vi "Auto Drive.vi"(0 "Ticks(Distance)":dbl=978.0 format="%#_13g", 1 "Swerve DevRef":T2[](array[typedef])=[{"DeviceStatus"={"status"=FALSE, "code"=0, "source"=""}, "Type"=enum."CAN", "PWM"={"PWM Channel"=enum."PWM 1", "DeadBand"={"Name"="", "maxPositivePwm"=0, "minPositivePwm"=0, "centerPwm"=0, "maxNegativePwm"=0, "minNegativePwm"=0, "angularRange"=0}}, "CAN"={"Device Number"=4, "SetOutput VI Ref"=variant(refnum<vi> refnum), "GetOutput VI Ref"=variant(refnum<vi> refnum), "Enable VI Ref"=variant(refnum<vi> refnum), "Disable VI Ref"=variant(refnum<vi> refnum), "Data"=variant(cluster{"Control Mode":enum8{"Percent VBus", "Speed", "Position", "Slave", "Unchanged / Invalid", "Voltage Compensation", "Current", "Motion Profile", "Motion Magic"}, "Encoder Initial Position":dbl, "MaxVout":dbl} {"Control Mode"=enum."Position", "Encoder Initial Position"=0.0, "MaxVout"=12.0})}, "Invert"=FALSE}, {"DeviceStatus"={"status"=FALSE, "code"=0, "source"=""}, "Type"=enum."CAN", "PWM"={"PWM Channel"=enum."PWM 1", "DeadBand"={"Name"="", "maxPositivePwm"=0, "minPositivePwm"=0, "centerPwm"=0, "maxNegativePwm"=0, "minNegativePwm"=0, "angularRange"=0}}, "CAN"={"Device Number"=8, "SetOutput VI Ref"=variant(refnum<vi> refnum), "GetOutput VI Ref"=variant(refnum<vi> refnum), "Enable VI Ref"=variant(refnum<vi> refnum), "Disable VI Ref"=variant(refnum<vi> refnum), "Data"=variant(cluster{"Control Mode":enum8{"Percent VBus", "Speed", "Position", "Slave", "Unchanged / Invalid", "Voltage Compensation", "Current", "Motion Profile", "Motion Magic"}, "Encoder Initial Position":dbl, "MaxVout":dbl} {"Control Mode"=enum."Position", "Encoder Initial Position"=0.0, "MaxVout"=12.0})}, "Invert"=FALSE}, {"DeviceStatus"={"status"=FALSE, "code"=0, "source"=""}, "Type"=enum."CAN", "PWM"={"PWM Channel"=enum."PWM 1", "DeadBand"={"Name"="", "maxPositivePwm"=0, "minPositivePwm"=0, "centerPwm"=0, "maxNegativePwm"=0, "minNegativePwm"=0, "angularRange"=0}}, "CAN"={"Device Number"=6, "SetOutput VI Ref"=variant(refnum<vi> refnum), "GetOutput VI Ref"=variant(refnum<vi> refnum), "Enable VI Ref"=variant(refnum<vi> refnum), "Disable VI Ref"=variant(refnum<vi> refnum), "Data"=variant(cluster{"Control Mode":enum8{"Percent VBus", "Speed", "Position", "Slave", "Unchanged / Invalid", "Voltage Compensation", "Current", "Motion Profile", "Motion Magic"}, "Encoder Initial Position":dbl, "MaxVout":dbl} {"Control Mode"=enum."Position", "Encoder Initial Position"=0.0, "MaxVout"=12.0})}, "Invert"=FALSE}, {"DeviceStatus"={"status"=FALSE, "code"=0, "source"=""}, "Type"=enum."CAN", "PWM"={"PWM Channel"=enum."PWM 1", "DeadBand"={"Name"="", "maxPositivePwm"=0, "minPositivePwm"=0, "centerPwm"=0, "maxNegativePwm"=0, "minNegativePwm"=0, "angularRange"=0}}, "CAN"={"Device Number"=2, "SetOutput VI Ref"=variant(refnum<vi> refnum), "GetOutput VI Ref"=variant(refnum<vi> refnum), "Enable VI Ref"=variant(refnum<vi> refnum), "Disable VI Ref"=variant(refnum<vi> refnum), "Data"=variant(cluster{"Control Mode":enum8{"Percent VBus", "Speed", "Position", "Slave", "Unchanged / Invalid", "Voltage Compensation", "Current", "Motion Profile", "Motion Magic"}, "Encoder Initial Position":dbl, "MaxVout":dbl} {"Control Mode"=enum."Position", "Encoder Initial Position"=0.0, "MaxVout"=12.0})}, "Invert"=FALSE}], 5 "Drive Angle":dbl=3.141592653589793, 7 "Start Power":dbl=0.2 format="%#_13g", 9 "Time Condition":u32=15000, 11 "error in":errorcluster, 12 "Wheel DevRef":T2[](array[typedef])=[{"DeviceStatus"={"status"=FALSE, "code"=0, "source"=""}, "Type"=enum."CAN", "PWM"={"PWM Channel"=enum."PWM 1", "DeadBand"={"Name"="", "maxPositivePwm"=0, "minPositivePwm"=0, "centerPwm"=0, "maxNegativePwm"=0, "minNegativePwm"=0, "angularRange"=0}}, "CAN"={"Device Number"=3, "SetOutput VI Ref"=variant(refnum<vi> refnum), "GetOutput VI Ref"=variant(refnum<vi> refnum), "Enable VI Ref"=variant(refnum<vi> refnum), "Disable VI Ref"=variant(refnum<vi> refnum), "Data"=variant(cluster{"Control Mode":enum8{"Percent VBus", "Speed", "Position", "Slave", "Unchanged / Invalid", "Voltage Compensation", "Current", "Motion Profile", "Motion Magic"}, "Encoder Initial Position":dbl, "MaxVout":dbl} {"Control Mode"=enum."Percent VBus", "Encoder Initial Position"=0.0, "MaxVout"=12.0})}, "Invert"=TRUE}, {"DeviceStatus"={"status"=FALSE, "code"=0, "source"=""}, "Type"=enum."CAN", "PWM"={"PWM Channel"=enum."PWM 1", "DeadBand"={"Name"="", "maxPositivePwm"=0, "minPositivePwm"=0, "centerPwm"=0, "maxNegativePwm"=0, "minNegativePwm"=0, "angularRange"=0}}, "CAN"={"Device Number"=7, "SetOutput VI Ref"=variant(refnum<vi> refnum), "GetOutput VI Ref"=variant(refnum<vi> refnum), "Enable VI Ref"=variant(refnum<vi> refnum), "Disable VI Ref"=variant(refnum<vi> refnum), "Data"=variant(cluster{"Control Mode":enum8{"Percent VBus", "Speed", "Position", "Slave", "Unchanged / Invalid", "Voltage Compensation", "Current", "Motion Profile", "Motion Magic"}, "Encoder Initial Position":dbl, "MaxVout":dbl} {"Control Mode"=enum."Percent VBus", "Encoder Initial Position"=0.0, "MaxVout"=12.0})}, "Invert"=TRUE}, {"DeviceStatus"={"status"=FALSE, "code"=0, "source"=""}, "Type"=enum."CAN", "PWM"={"PWM Channel"=enum."PWM 1", "DeadBand"={"Name"="", "maxPositivePwm"=0, "minPositivePwm"=0, "centerPwm"=0, "maxNegativePwm"=0, "minNegativePwm"=0, "angularRange"=0}}, "CAN"={"Device Number"=5, "SetOutput VI Ref"=variant(refnum<vi> refnum), "GetOutput VI Ref"=variant(refnum<vi> refnum), "Enable VI Ref"=variant(refnum<vi> refnum), "Disable VI Ref"=variant(refnum<vi> refnum), "Data"=variant(cluster{"Control Mode":enum8{"Percent VBus", "Speed", "Position", "Slave", "Unchanged / Invalid", "Voltage Compensation", "Current", "Motion Profile", "Motion Magic"}, "Encoder Initial Position":dbl, "MaxVout":dbl} {"Control Mode"=enum."Percent VBus", "Encoder Initial Position"=0.0, "MaxVout"=12.0})}, "Invert"=FALSE}, {"DeviceStatus"={"status"=FALSE, "code"=0, "source"=""}, "Type"=enum."CAN", "PWM"={"PWM Channel"=enum."PWM 1", "DeadBand"={"Name"="", "maxPositivePwm"=0, "minPositivePwm"=0, "centerPwm"=0, "maxNegativePwm"=0, "minNegativePwm"=0, "angularRange"=0}}, "CAN"={"Device Number"=1, "SetOutput VI Ref"=variant(refnum<vi> refnum), "GetOutput VI Ref"=variant(refnum<vi> refnum), "Enable VI Ref"=variant(refnum<vi> refnum), "Disable VI Ref"=variant(refnum<vi> refnum), "Data"=variant(cluster{"Control Mode":enum8{"Percent VBus", "Speed", "Position", "Slave", "Unchanged / Invalid", "Voltage Compensation", "Current", "Motion Profile", "Motion Magic"}, "Encoder Initial Position":dbl, "MaxVout":dbl} {"Control Mode"=enum."Percent VBus", "Encoder Initial Position"=0.0, "MaxVout"=12.0})}, "Invert"=FALSE}]) -> (15 "error out":errorcluster)   [LabVIEW 2016]
uses:
  <vilib>/Rock Robotics/WPI/MotorControl/WPI_MotorControlDeviceRef.ctl
  <vilib>/Rock Robotics/WPI/MotorControl/WPI_MotorControlType.ctl
  <vilib>/Rock Robotics/SystemInterfaces/DIO/FPGA_DIOPWMChannel.ctl
  <vilib>/Rock Robotics/WPI/PWM/WPI_PWMDeadband.ctl
  <vilib>/addons/control/pid/pid.llb/PID (DBL).vi
  <vilib>/addons/control/pid/NI_PID_pid.lvlib
panel:
  out "Setpoint":dbl(graph)=-2640.109929651602
  out "Wheel 1":dbl(graph)=-0.2756567273293147
  out "Wheel 3 Chart":dbl(graph)=0.2756567273293147
  out "Z":dbl(graph)=0.38894343516186153
  out "Difference":dbl(graph)=18.0
  in  "output range":cluster{"output high":dbl, "output low":dbl}={"output high"=1.0, "output low"=-1.0} {"output low" format="%.2f"; "output high" format="%.2f"}
  in  "PID gains Rotational Correction":T1={"proportional gain (Kc)"=2.5e-05, "integral time (Ti, min)"=0.008, "derivative time (Td, min)"=0.0} {"derivative time (Td, min)" format="%.3f"; "integral time (Ti, min)" format="%.6f"; "proportional gain (Kc)" format="%.9f"}
  # ".000025 p"
  # ".008 i"
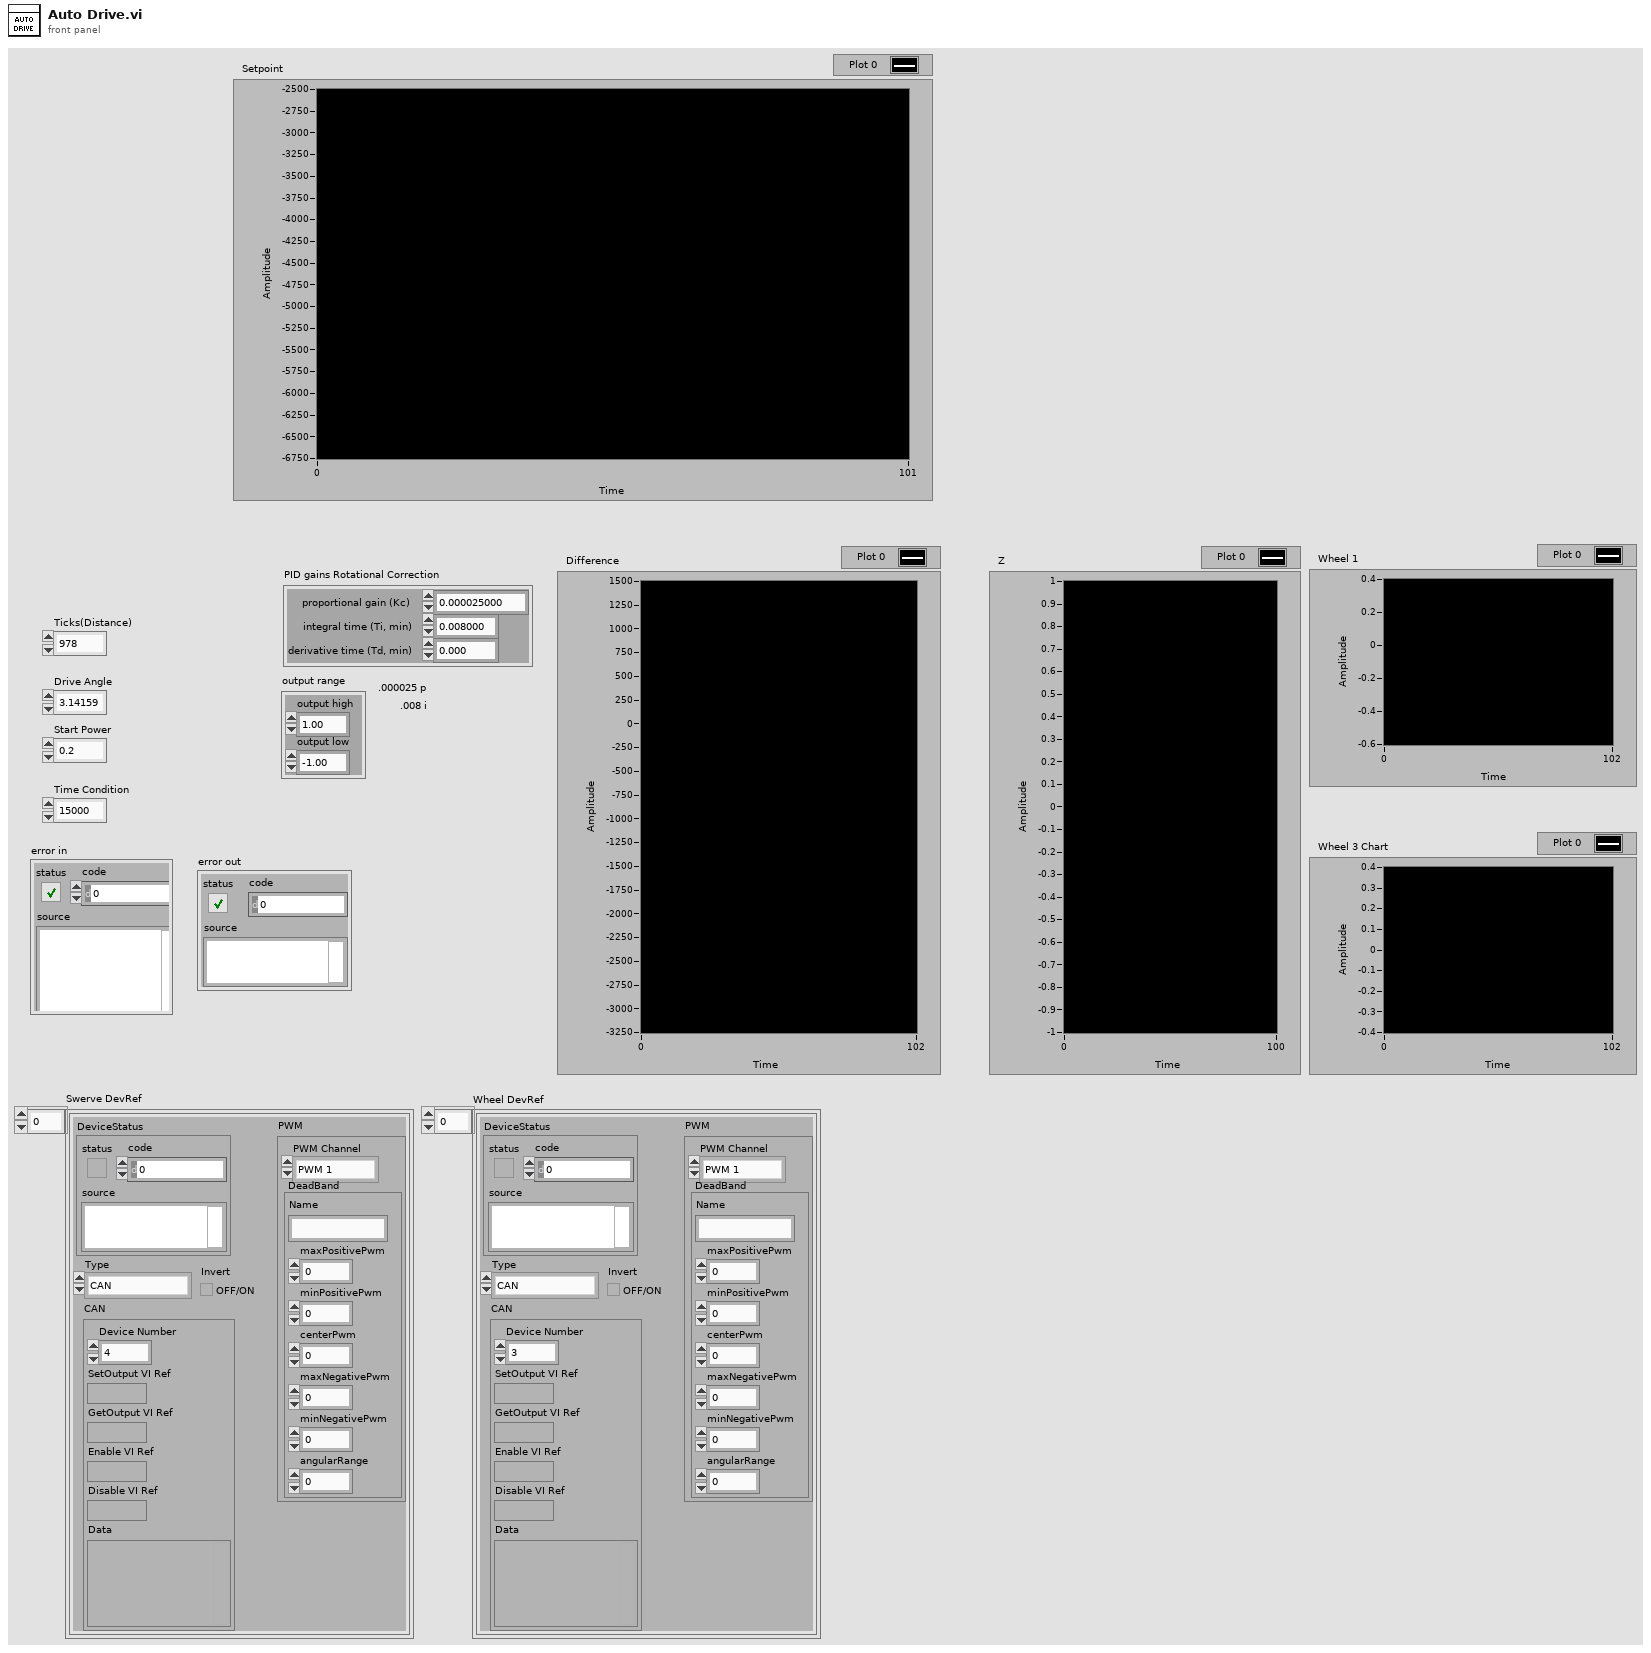
[diagram p1: front panel]
types:
  T1 = cluster{"proportional gain (Kc)":dbl, "integral time (Ti, min)":dbl, "derivative time (Td, min)":dbl}
  T2 = typedef "WPI_MotorControlDeviceRef.ctl" = cluster{"DeviceStatus":errorcluster, "Type":T3, "PWM":cluster{"PWM Channel":T4, "DeadBand":T5}, "CAN":cluster{"Device Number":u8, "SetOutput VI Ref":variant, "GetOutput VI Ref":variant, "Enable VI Ref":variant, "Disable VI Ref":variant, "Data":variant}, "Invert":bool}
  T3 = typedef "WPI_MotorControlType.ctl" = enum16{"PWM", "CAN"}
  T4 = typedef "FPGA_DIOPWMChannel.ctl" = enum8{"PWM 0", "PWM 1", "PWM 2", "PWM 3", "PWM 4", "PWM 5", "PWM 6", "PWM 7", "PWM 8", "PWM 9", "PWM MXP 0", "PWM MXP 1", "PWM MXP 2", "PWM MXP 3", "PWM MXP 4", "PWM MXP 5", "PWM MXP 6", "PWM MXP 7", "PWM MXP 8", "PWM MXP 9", "Invalid"}
  T5 = typedef "WPI_PWMDeadband.ctl" = cluster{"Name":string, "maxPositivePwm":i32, "minPositivePwm":i32, "centerPwm":i32, "maxNegativePwm":i32, "minNegativePwm":i32, "angularRange":u16}
  T6 = typedef "WPI_CANTalonSRX_GlobalStatus.ctl" = cluster{"Applied Throttle":dbl, "Module Enabled":bool, "CAN Error":errorcluster, "Closed Loop Error":dbl, "Forward Limit Switch Closed":bool, "Reverse Limit Switch Closed":bool, "Sensor Position":dbl, "Sensor Velocity":dbl, "Current":dbl, "Sticky Fault - Over Temp":bool, "Sticky Fault - Under Voltage":bool, "Sticky Fault - Forward Limit":bool, "Sticky Fault - Reverse Limit":bool, "Sticky Fault - Forward Soft Limit":bool, "Sticky Fault - Reverse Soft Limit":bool, "Brake is Enabled":bool, "Encoder Position":dbl, "Encoder Velocity":dbl, "Encoder Index Count":dbl, "Encoder A Pin State":bool, "Encoder B Pin State":bool, "Encoder Index Pin State":bool, "Analog In":dbl, "Analog In Velocity":dbl, "Temperature (C)":dbl, "Battery Voltage":dbl, "Control 5 Is Supported":bool, "Current Profile Slot Select":dbl, "Pos Div 8":bool, "Vel Div 4":bool, "Pulse Width Position":i32, "Pulse Width Velocity":i32, "Pulse Width Rise To Rise (us)":i32, "Pulse Width Rise To Fall (us)":i32, "Mot Prof Active Is Under Run":bool, "Mot Prof Active Has Under Run":bool, "Mot Prof Active Is Last":bool, "Mot Prof Active Velocity Only":bool, "Mot Prof Active Is Valid":bool, "Mot Prof Buffer Is Full":bool, "Mot Prof Active Profile Slot Select":i32, "Mot Prof NextID":i32, "Mot Prof Count":i32, "Mot Prof Active Velocity":dbl, "Mot Prof Active Position":dbl, "Mot Prof Output Enable":i32}
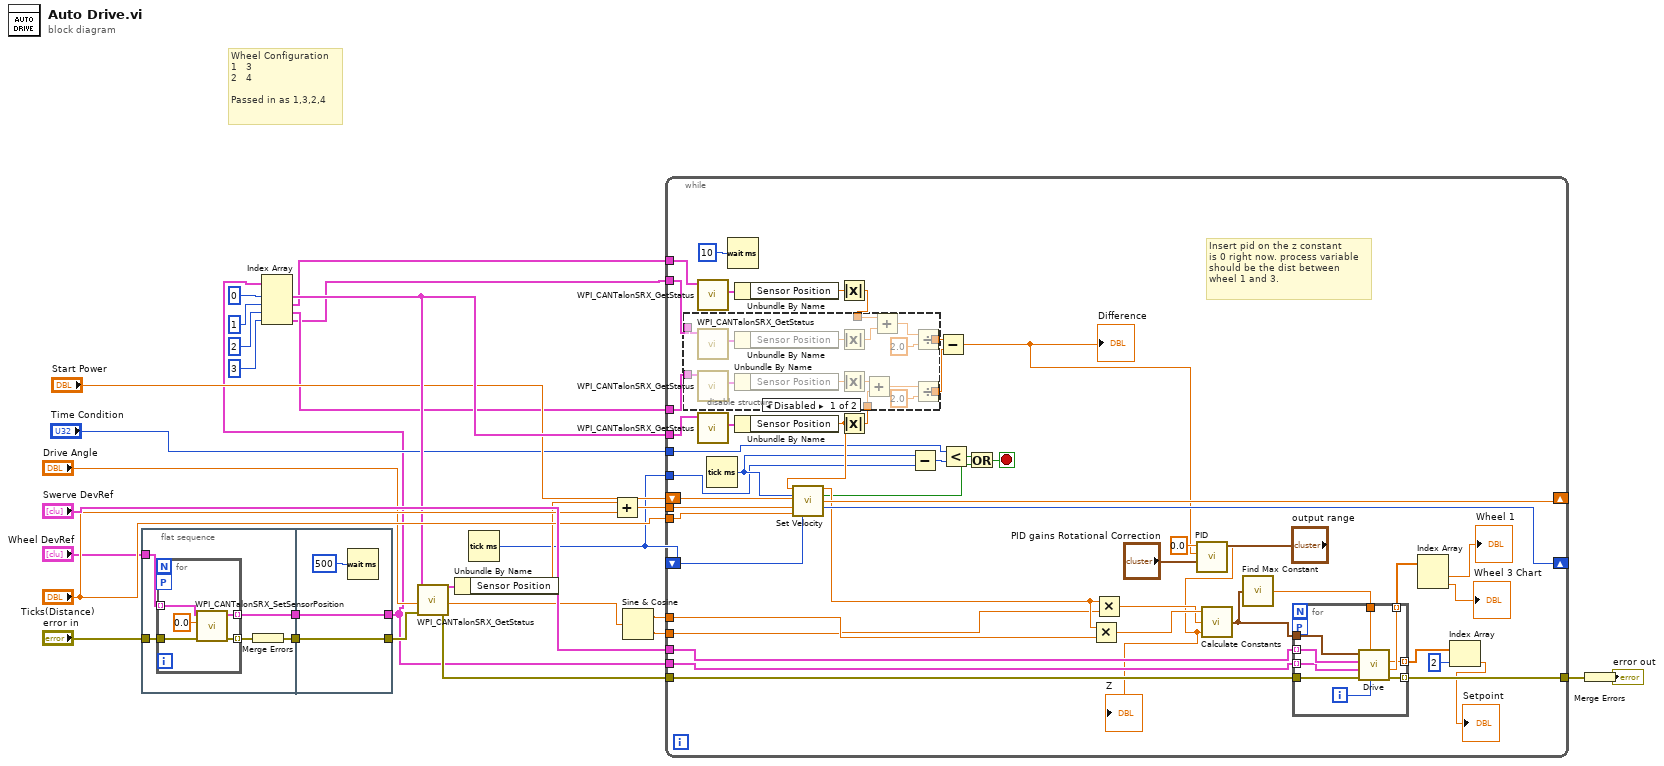
[diagram p0: block diagram]
diagram:
  # "Wheel Configuration\n1   3\n2   4\n\nPassed in as 1,3,2,4"
  n1 = flat-sequence {
    tunnel: "Wheel DevRef" -> [w33]
    tunnel: "error in" -> [w31]
    tunnel: [w32] -> w3
    tunnel: [w29] -> w2
    tunnel: [w40] -> w11
    tunnel: [w41] -> w1
    tunnel: w3 -> [w41]
    tunnel: w2 -> [w40]
    frame #0 {
      n2 = for {
        tunnel: w33 -> [w38] mode=indexing
        tunnel: [w36] -> w32 mode=indexing
        workers-P: _ -> [_]
        tunnel: w31 -> [w35]
        tunnel: [w34] -> w30 mode=indexing
        n3 = call <vilib>:"WPI_CANTalonSRX_SetSensorPosition.vi"("error in (no error)"=w35, "New Sensor Position"=0.0, "CAN Talon SRX Ref"=w38) -> ("error out"=w34:errorcluster, "CAN Talon SRX Ref"=w36:T2)  [unwired: 7 in]
      }
      n4 = Merge Errors(w30) -> (w29:errorcluster)
    }
    frame #1 {
      n5 = Wait (ms)(milliseconds to wait=u32 500) -> ()  [unwired: 1 out]
    }
  }
  n6 = Index Array(array=w1, index #1=0 ("index"), index #2=1 ("index"), index #3=2 ("index"), index #4=3 ("index")) -> (element #1=w23:T2, element #2=w13:T2, element #3=w7:T2, element #4=w6:T2)
  n7 = call <vilib>:"WPI_CANTalonSRX_GetStatus.vi"("error in (no error)"=w11, "CAN Talon SRX Ref"=w23) -> ("error out"=w10:errorcluster, "Talon SRX Status"=w27:T6)  [unwired: 7 in, 1 out]
  n8 = Unbundle By Name(w27) -> ("Sensor Position"=w25:dbl)
  n9 = Tick Count (ms)() -> (millisecond timer value=w4:u32)
  n10 = Add(x=w25, y="Ticks(Distance)") -> (x+y=w24:dbl)
  n11 = Sine & Cosine(0:"Drive Angle") -> (1:w18:dbl, 2:w17:dbl)
  n12 = while {
    tunnel: w10 -> [w83]
    tunnel: [w84] -> w21
    tunnel: "Swerve DevRef" -> [w89]
    tunnel: w24 -> [w86]
    tunnel: w1 -> [w88]
    tunnel: w23 -> [w87]
    tunnel: "Ticks(Distance)" -> [w85]
    shift-right: [w81] -> _
    shift-left: "Start Power" -> [w82]
    shift-right: [w80] -> _
    shift-left: w4 -> [w46]
    tunnel: w18 -> [w74]
    tunnel: w17 -> [w73]
    tunnel: w13 -> [w71]
    tunnel: w7 -> [w60]
    tunnel: w6 -> [w58]
    tunnel: "Time Condition" -> [w51]
    tunnel: w4 -> [w42]
    stop <- w50 stop-if-true
    # "Insert pid on the z constant\nis 0 right now. process variable\nshould be the dist between \nwheel 1 and 3."
    n13 = call <vilib>:"WPI_CANTalonSRX_GetStatus.vi"("CAN Talon SRX Ref"=w71) -> ("Talon SRX Status"=w72:T6)  [unwired: 8 in, 2 out]
    n14 = call <vilib>:"WPI_CANTalonSRX_GetStatus.vi"("CAN Talon SRX Ref"=w87) -> ("Talon SRX Status"=w78:T6)  [unwired: 8 in, 2 out]
    n15 = Tick Count (ms)() -> (millisecond timer value=w47:u32)
    n16 = Wait (ms)(milliseconds to wait=u32 10) -> ()  [unwired: 1 out]
    n17 = Unbundle By Name(w72) -> ("Sensor Position"=w70:dbl)
    n18 = Unbundle By Name(w78) -> ("Sensor Position"=w69:dbl)
    n19 = call "Set Velocity.vi"("Process Variable(x)"=w69, "Current TIme"=w47, "Current Power"=w82, "Setpoint(end)"=w86, "Total Distance"=w85, "Last Time Input"=w46) -> ("Coerced Motor power"=w79:dbl, "End Loop?"=w54:bool, "Non-Coerced Motor Power"=w81:dbl, "Last Time Output"=w80:u32)  [unwired: 6 in]
    n20 = Absolute Value(x=w70) -> (abs(x)=w57:dbl)
    n21 = Absolute Value(x=w69) -> (abs(x)=w59:dbl)
    n22 = disable-structure shown="Disabled" {
      disable-tunnel: w60 -> [w104 _]
      disable-tunnel: w59 -> [w100 w107]
      disable-tunnel: w58 -> [w98 _]
      disable-tunnel: w57 -> [w96 w106]
      disable-tunnel: [w92 w107] -> w56
      disable-tunnel: [w91 w106] -> w55
      frame Disabled {
        n23 = call <vilib>:"WPI_CANTalonSRX_GetStatus.vi"("CAN Talon SRX Ref"=w98) -> ("Talon SRX Status"=w97:T6)  [unwired: 8 in, 2 out]
        n24 = call <vilib>:"WPI_CANTalonSRX_GetStatus.vi"("CAN Talon SRX Ref"=w104) -> ("Talon SRX Status"=w105:T6)  [unwired: 8 in, 2 out]
        n25 = Unbundle By Name(w97) -> ("Sensor Position"=w99:dbl)
        n26 = Unbundle By Name(w105) -> ("Sensor Position"=w103:dbl)
        n27 = Absolute Value(x=w99) -> (abs(x)=w90:dbl)
        n28 = Absolute Value(x=w103) -> (abs(x)=w101:dbl)
        n29 = Add(x=w101, y=w100) -> (x+y=w102:dbl)
        n30 = Add(x=w96, y=w90) -> (x+y=w95:dbl)
        n31 = Divide(x=w95, y=2.0) -> (x/y=w91:dbl)
        n32 = Divide(x=w102, y=2.0) -> (x/y=w92:dbl)
      }
      frame Enabled {
      }
    }
    n33 = Subtract(x=w47, y=w42) -> (x-y=w48:u32)
    n34 = Subtract(x=w55, y=w56) -> (x-y=w53:dbl)
    "Difference" <- w53
    n35 = Less?(x=w51, y=w48) -> (x < y?=w49:bool)
    n36 = Or(x=w49, y=w54) -> (x .or. y?=w50:bool)
    n37 = Multiply(x=w79, y=w74) -> (x*y=w77:dbl)
    n38 = Multiply(x=w79, y=w73) -> (x*y=w76:dbl)
    n39 = call-poly <vilib>:"PID.vi"("output range"="output range", "PID gains"="PID gains Rotational Correction", "process variable"=w53, "setpoint"=0.0) -> ("output"=w63:dbl)  [unwired: 6 in, 1 out]
    "Z" <- w63
    n40 = call "Calculate Constants.vi"("Z"=w63, "Y"=w76, "X"=w77) -> ("constants cluster"=w64:cluster{"a":dbl, "b":dbl, "c":dbl, "d":dbl})
    n41 = call "Find Max Constant.vi"("constants"=w64) -> ("Max or 1"=w65:dbl)
    n42 = for {
      tunnel: w64 -> [w116]
      tunnel: w89 -> [w115] mode=indexing
      tunnel: w88 -> [w114] mode=indexing
      workers-P: _ -> [_]
      tunnel: [w112] -> w84 mode=indexing
      tunnel: w83 -> [w111]
      tunnel: w65 -> [w110]
      tunnel: [w109] -> w52 mode=indexing
      tunnel: [w108] -> w45 mode=indexing
      i -> [w113]
      n43 = call "Drive.vi"("Index"=w113, "Max Speed or 1"=w110, "error in"=w111, "Wheel DevRef"=w114, "Swerve DevRef"=w115, "constants"=w116) -> ("error out"=w112:errorcluster, "Wheel Speed"=w109:dbl, "Setpoint"=w108:dbl)  [unwired: 1 in, 2 out]
    }
    n44 = Index Array(array=w52) -> (element #1=→"Wheel 1":dbl, element #2=→"Wheel 3 Chart":dbl)  [unwired: 2 in]
    n45 = Index Array(array=w45, index=2) -> (element=→"Setpoint":dbl)
  }
  n46 = Merge Errors(w21) -> (→"error out":errorcluster)
